vi "ConfigurationDialog.vi"(2 "Format In":cluster{"Rate":i32, "Bits":i32, "Channels":u32}, 3 "Buffer Config In":T1) -> (0 "Format Out":cluster{"Rate":i32, "Bits":i32, "Channels":u32}, 1 "Buffer Config Out":T1)   [LabVIEW 2016]
panel:
  in  "Cancel Button":bool
  in  "OK Button":bool
  in  "Format":cluster{"Rate":i32, "Bits":i32, "Channels":u32}
  in  "Buffer Config":T1
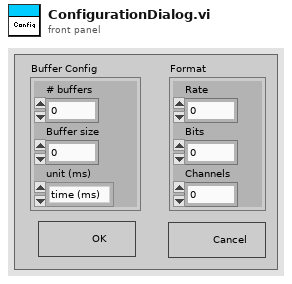
[diagram p1: front panel]
types:
  T1 = cluster{"# buffers":i32, "Buffer size":i32, "unit (ms)":enum16{"time (ms)", "Samples"}}
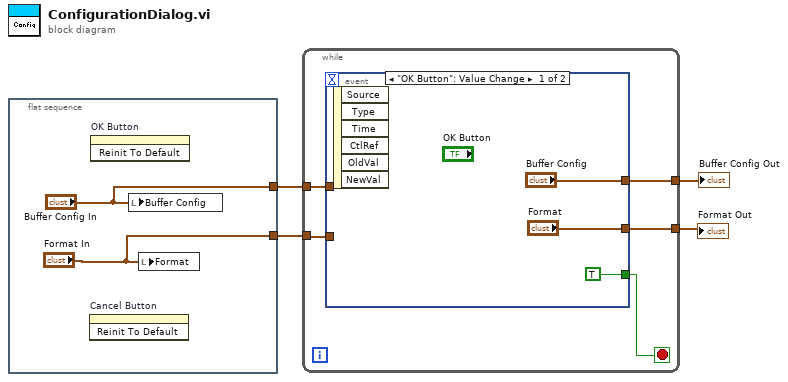
[diagram p0: block diagram]
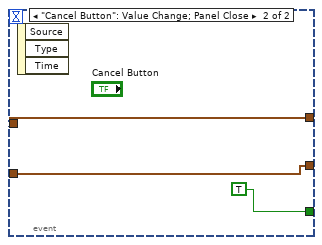
[diagram p2: hidden frame]
diagram:
  n1 = flat-sequence {
    tunnel: ["Format In"] -> w2
    tunnel: ["Buffer Config In"] -> w1
    frame #0 {
      n2 = invoke on="Cancel Button" class="Bool (strict)" method="Reinit To Default"() -> ()  [unwired: 3 in, 3 out]
      n3 = invoke on="OK Button" class="Bool (strict)" method="Reinit To Default"() -> ()  [unwired: 3 in, 3 out]
      n4 = local write "Buffer Config"("Buffer Config In") -> ()
      n5 = local write "Format"("Format In") -> ()
    }
  }
  n6 = while {
    tunnel: [w10] -> w4
    tunnel: [w9] -> w3
    tunnel: w2 -> [w8]
    tunnel: w1 -> [w7]
    stop <- w11 stop-if-true
    n7 = event shown="[0] \"OK Button\": Value Change" {
      selector: _ -> [_ _]
      dyn-events: _ -> [_ _]
      timeout: _ -> [_ _]
      tunnel: [TRUE TRUE] -> w11
      tunnel: ["Buffer Config" w15] -> w10
      tunnel: ["Format" w16] -> w9
      tunnel: w8 -> [_ w16]
      tunnel: w7 -> [_ w15]
      event "OK Button": Value Change {
        n8 = event-data() -> ()  [unwired: 1 in, 6 out]
      }
      event "Cancel Button": Value Change; Panel Close {
        n9 = event-data() -> ()  [unwired: 1 in, 3 out]
      }
    }
  }
  "Format Out" <- w3
  "Buffer Config Out" <- w4
